vi "Autodiscover Group Async.vi"(10 "Discovery":T4, 11 "RemoteDataService in":refnum<class "RemoteDataService.lvclass">) -> ()   [LabVIEW 2020, in "Vecto.lvlib" / "RemoteDataService.lvclass"]
uses:
  RemoteDataService.lvclass
  proto/Discovery/Data.ctl
  proto/Service/Data.ctl
  proto/ServiceType/Enumeration.ctl
  Publish Config Response.ctl
  Publish Config Response Group.ctl
  Publish Config.ctl
  RemoteDataService.lvclass/RemoteDataService.ctl
  Group Info.ctl
  Channel Init.ctl
  Vecto.lvlib
  proto/ServiceType/ServiceType.lvlib
  <vilib>/httpClient/LabVIEWHTTPClient.lvlib
  Group Config/Group Config.lvclass
  ChannelService/ChannelService.lvclass
  proto/Service/Service.lvlib
  proto/Discovery/Discovery.lvlib
panel:
  out "Publish Config Response":T1
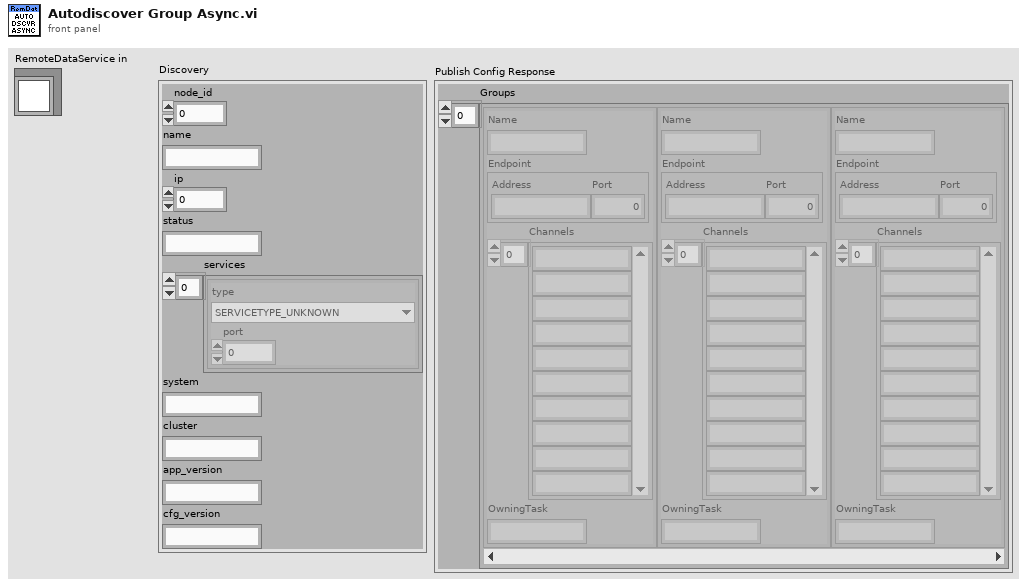
[diagram p1: front panel]
types:
  T1 = typedef "Vecto.lvlib/Publish Config Response.ctl" = cluster{"Groups":T2[]}
  T2 = typedef "Vecto.lvlib/Publish Config Response Group.ctl" = cluster{"Name":string, "Endpoint":T3, "Channels":string[], "OwningTask":string}
  T3 = typedef "Vecto.lvlib/Publish Config.ctl" = cluster{"Address":string, "Port":u16}
  T4 = typedef "Discovery.lvlib/Data.ctl" = cluster{"node_id":u32, "name":string, "ip":u32, "status":string, "services":T5[], "system":string, "cluster":string, "app_version":string, "cfg_version":string}
  T5 = typedef "Service.lvlib/Data.ctl" = cluster{"type":T6, "port":i32}
  T6 = typedef "ServiceType.lvlib/Enumeration.ctl" = enum16{"SERVICETYPE_UNKNOWN", "SERVICETYPE_TCPSERVER", "SERVICETYPE_HTTPSERVER"}
  T7 = typedef "Vecto.lvlib/Group Info.ctl" = cluster{"System":string, "Cluster":string, "Node":string, "Task":string, "Name":string}
  T8 = typedef "Vecto.lvlib/Channel Init.ctl" = cluster{"Name":string, "Resource":string}
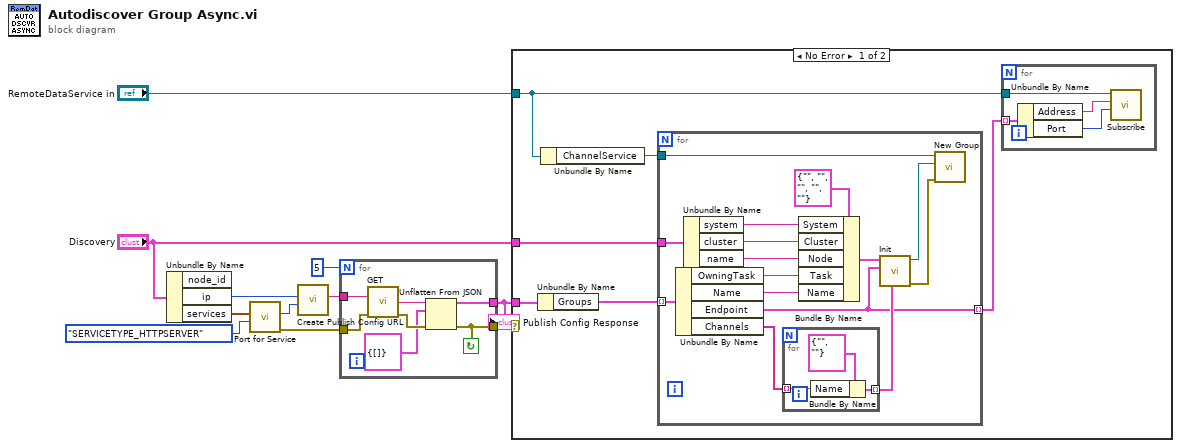
[diagram p0: block diagram]
diagram:
  n1 = Unbundle By Name("Discovery") -> ("ip"=w9:u32, "services"=w11:T5[])  [unwired: 1 out]
  n2 = call "Port for Service.vi"("type"=Enumeration."SERVICETYPE_HTTPSERVER", "services"=w11) -> ("error out"=w6:errorcluster, "port"=w8:i32)  [unwired: 8 in]
  n3 = call "Create Publish Config URL.vi"("port"=w8, "ip"=w9) -> ("String"=w7:string)  [unwired: 9 in]
  n4 = for {
    N: 5 -> [_]
    tunnel: w7 -> [w18]
    tunnel: w6 -> [w17]
    tunnel: [w13] -> w3
    tunnel: [w12] -> w4
    stop <- w12 continue-if-true
    n5 = call <vilib>:"GET.vi"("url"=w18, "error in (no error)"=w17) -> ("body"=w16:string, "error out"=w15:errorcluster)  [unwired: 10 in, 2 out]
    n6 = Unflatten From JSON(JSON string=w16, type and defaults=T1 {"Groups"=[]} ("Publish Config Response"), error in (no error)=w15) -> (value=w13:T1, error out=w12:errorcluster)  [unwired: 4 in]
  }
  "Publish Config Response" <- w3
  n7 = case shown="No Error" w4 {
    tunnel: w3 -> [w24 _]
    tunnel: "RemoteDataService in" -> [w20 _]
    tunnel: "Discovery" -> [w21 _]
    frame No Error {
      n8 = Unbundle By Name(w24) -> ("Groups"=w23:T2[])
      n9 = Unbundle By Name(w20) -> ("ChannelService"=w22:refnum<class "ChannelService.lvclass">)
      n10 = for {
        tunnel: w23 -> [w43] mode=indexing
        tunnel: w22 -> [w32]
        tunnel: w21 -> [w41]
        tunnel: [w29] -> w19 mode=indexing
        n11 = Unbundle By Name(w43) -> ("OwningTask"=w36:string, "Name"=w35:string, "Endpoint"=w29:T3, "Channels"=w34:string[])
        n12 = Unbundle By Name(w41) -> ("system"=w39:string, "cluster"=w38:string, "name"=w37:string)
        n13 = for {
          tunnel: w34 -> [w45] mode=indexing
          tunnel: [w44] -> w33 mode=indexing
          n14 = Bundle By Name(cluster=T8 {"Name"="", "Resource"=""} ("Channel Init"), "Name"=w45) -> (w44:T8)
        }
        n15 = Bundle By Name(cluster=T7 {"System"="", "Cluster"="", "Node"="", "Task"="", "Name"=""} ("Group Info"), "System"=w39, "Cluster"=w38, "Node"=w37, "Task"=w36, "Name"=w35) -> (w40:T7)
        n16 = call "Init.vi"("Channels"=w33, "Publish Config (None)"=w29, "Group Info"=w40) -> ("error out"=w30:errorcluster, "Group Config out"=w31:refnum<class "Group Config.lvclass">)  [unwired: 7 in]
        n17 = call "New Group.vi"("error in (no error)"=w30, "Group Config"=w31, "ChannelService in"=w32) -> ()  [unwired: 6 in, 3 out]
      }
      n18 = for {
        tunnel: w20 -> [w28]
        tunnel: w19 -> [w27] mode=indexing
        n19 = Unbundle By Name(w27) -> ("Address"=w26:string, "Port"=w25:u16)
        n20 = call "Subscribe.vi"("Multicast Port"=w25, "Multicast Address"=w26, "RemoteDataService in"=w28) -> ()  [unwired: 7 in, 2 out]
      }
    }
    frame Error {
    }
  }
